vi "Rundenzeit.vi"(11 "Startlinie":bool) -> (3 "Rundenzeiten":dbl[](array[numeric])=[inf, inf, inf, inf, inf, inf, inf, inf])   [LabVIEW 2016]
panel:
  # "Minimum"
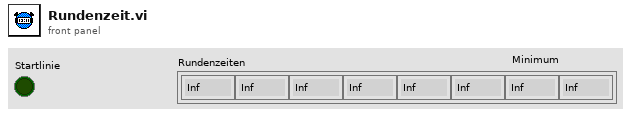
[diagram p1: front panel]
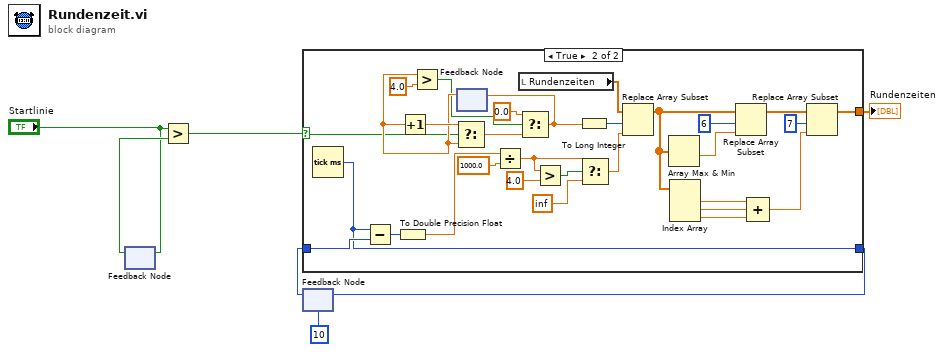
[diagram p0: block diagram]
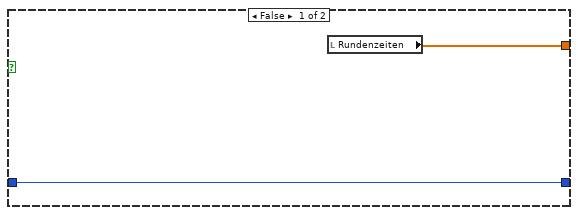
[diagram p2: hidden frame]
diagram:
  n1 = feedback #1() -> (w5:bool)  [unwired: 1 in]
  n2 = feedback-in #1("Startlinie") -> ()
  n3 = Greater?(x="Startlinie", y=w5) -> (0:w1:bool)
  n4 = feedback #2(u32 10 ("millisecond timer value")) -> (w6:u32)
  n5 = case shown="True" w1 {
    selector: w1 -> [_ w29]
    tunnel: [w9 w36] -> w7
    tunnel: w6 -> [w9 w39]
    tunnel: [w8 w17] -> w3
    frame False {
      n6 = local read "Rundenzeiten"() -> (w8:dbl[])
    }
    frame True {
      n7 = Tick Count (ms)() -> (millisecond timer value=w36:u32)
      n8 = Subtract(x=w36, y=w39) -> (x-y=w24:u32)
      n9 = To Double Precision Float(number=w24) -> (double precision float=w38:dbl)
      n10 = feedback #3() -> (w32:dbl)  [unwired: 1 in]
      n11 = Increment(x=w32) -> (x+1=w34:dbl)
      n12 = Greater?(x=w32, y=4.0) -> (0:w31:bool)
      n13 = Select(t=w34, s=w29, f=w32) -> (s? t:f=w33:dbl)
      n14 = Divide(x=w38, y=1000.0) -> (x/y=w21:dbl)
      n15 = local read "Rundenzeiten"() -> (w35:dbl[])
      n16 = Select(t=0.0, s=w31, f=w33) -> (s? t:f=w26:dbl)
      n17 = feedback-in #3(w26) -> ()
      n18 = Greater?(x=w21, y=4.0) -> (0:w22:bool)
      n19 = To Long Integer(number=w26) -> (32bit integer=w27:i32)
      n20 = Select(t=w21, s=w22, f=inf) -> (s? t:f=w20:dbl)
      n21 = Replace Array Subset(array=w35, new element=w20, index=w27) -> (w14:dbl[])
      n22 = Array Max & Min(array=w14) -> (min value=w15:dbl)  [unwired: 3 out]
      n23 = Index Array(array=w14) -> (element #1=w13:dbl, element #2=w12:dbl, element #3=w11:dbl)  [unwired: 3 in]
      n24 = Replace Array Subset(array=w14, new element=w15, index=6) -> (w18:dbl[])
      n25 = Compound Arithmetic op=ADD(w13, w12, w11) -> (w10:dbl)
      n26 = Replace Array Subset(array=w18, new element=w10, index=7) -> (w17:dbl[])
    }
  }
  "Rundenzeiten" <- w3
  n27 = feedback-in #2(w7) -> ()
